vi "update_dict_HIS_DAT_update.vi"(8 "error in (no error)":errorcluster, 10 "type":string, 11 "dict of HIS IN":variant) -> (0 "error out":errorcluster, 3 "dict of HIS OUT":variant)   [LabVIEW 2015]
uses:
  cluster_template.ctl
  Classes/DATA/HIS/HIS.lvclass
  Classes/DATA/HIS/HIS.lvclass/HIS.ctl
  Classes/DATA/DATA.lvclass/DATA.ctl
  Classes/DATA/DATA.lvclass
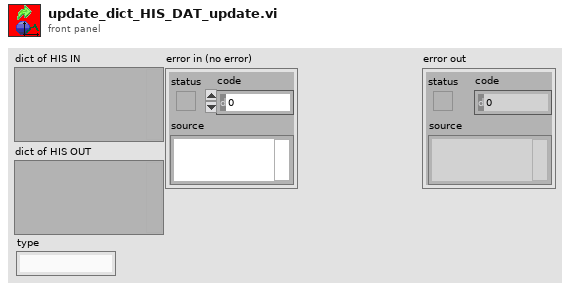
[diagram p1: front panel]
types:
  T1 = typedef "cluster_template.ctl" = cluster{"HIS.lvclass":refnum<class "HIS.lvclass">, "selector":refnum<vi>, "HIS graph":refnum<vi>, "DAT graph":refnum<vi>, "path":refnum<vi>, "path MAIN":refnum<vi>, "#":refnum<vi>, "unsel Graph":refnum<vi>, "DATgraph":refnum<vi>}
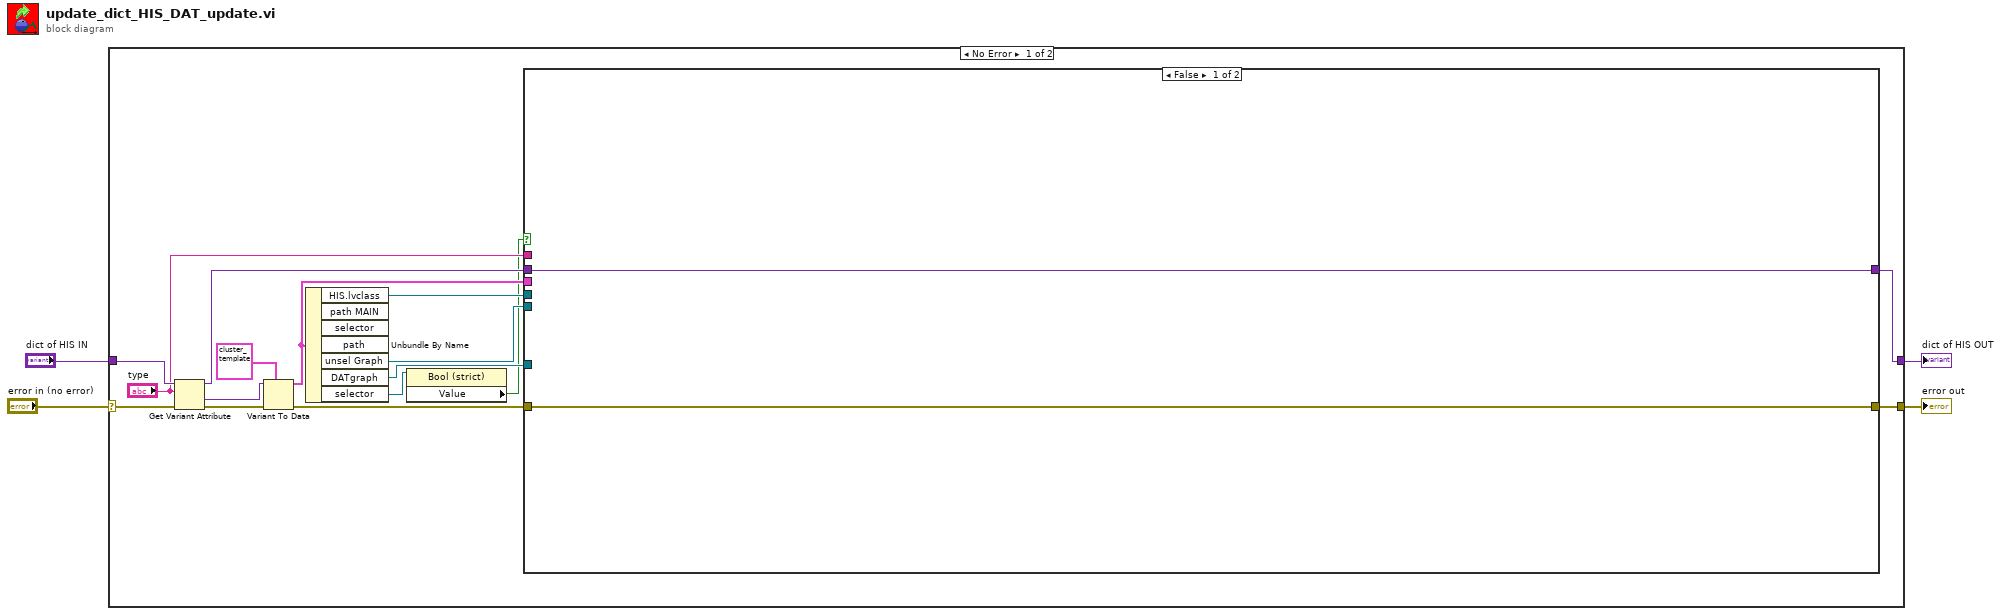
[diagram p0: block diagram]
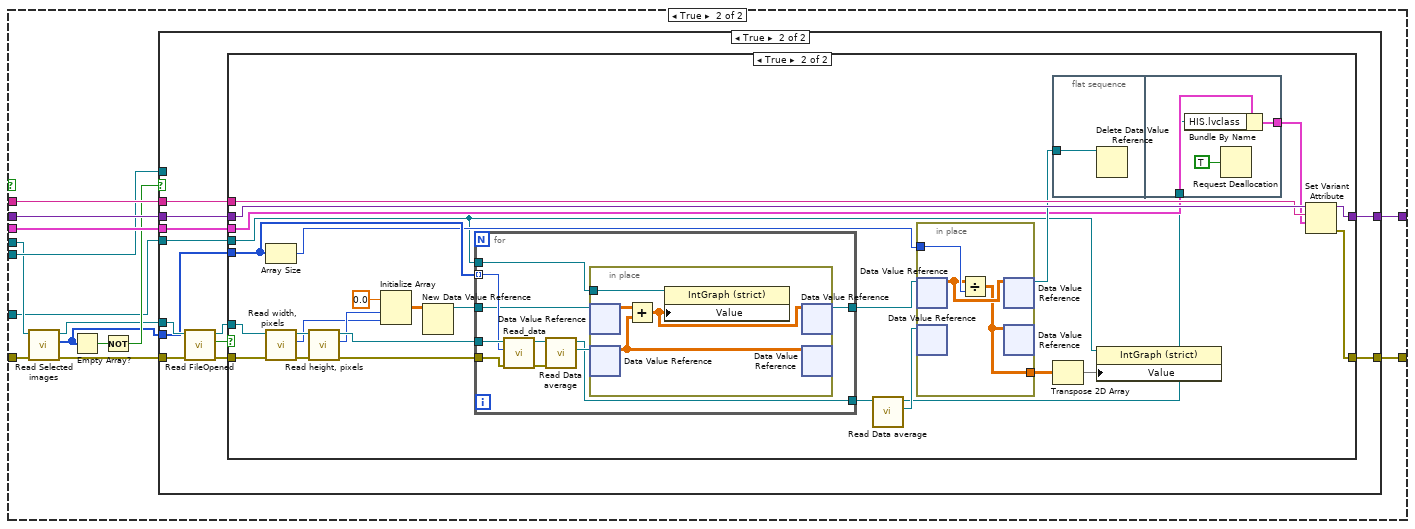
[diagram p2: hidden frame]
diagram:
  n1 = case shown="No Error" "error in (no error)" {
    selector: "error in (no error)" -> [w19 w103]
    tunnel: "dict of HIS IN" -> [w20 w102]
    tunnel: [w14 w102] -> w3
    tunnel: [w10 w103] -> w2
    frame No Error {
      n2 = Get Variant Attribute(Variant=w20, name="type", error in=w19) -> (duplicate Variant=w13:variant, value=w18:variant, error out=w17:errorcluster)  [unwired: 1 in, 1 out]
      n3 = Variant To Data(error in=w17, type=T1 {"HIS.lvclass"=refnum, "selector"=refnum, "HIS graph"=refnum, "DAT graph"=refnum, "path"=refnum, "path MAIN"=refnum, "#"=refnum, "unsel Graph"=refnum, "DATgraph"=refnum} ("output cluster"), Variant=w18) -> (data=w15:T1, error out=w9:errorcluster)
      n4 = Unbundle By Name(w15) -> ("HIS.lvclass"=w8:refnum<class "HIS.lvclass">, "unsel Graph"=w11:refnum<vi>, "DATgraph"=w7:refnum<vi>, "selector"=w6:refnum<vi>)  [unwired: 3 out]
      n5 = property class="Bool (strict)"(reference=w6) -> ("Value"=w5:bool)  [unwired: 1 in, 2 out]
      n6 = case shown="False" w5 {
        tunnel: w15 -> [_ w36]
        tunnel: [w22 w35] -> w14
        tunnel: w13 -> [w22 w34]
        tunnel: "type" -> [_ w33]
        tunnel: w11 -> [_ w32]
        tunnel: [w21 w31] -> w10
        tunnel: w9 -> [w21 w30]
        tunnel: w8 -> [_ w29]
        tunnel: w7 -> [_ w23]
        frame False {
        }
        frame True {
          n7 = call "Read Selected images.vi"("error in (no error)"=w30, "HIS in"=w29) -> ("error out"=w26:errorcluster, "Selected images"=w25:i32[], "HIS out"=w24:refnum<class "HIS.lvclass">)  [unwired: 7 in]
          n8 = Empty Array?(array=w25) -> (empty?=w28:bool)
          n9 = Not(x=w28) -> (.not. x?=w27:bool)
          n10 = case shown="True" w27 {
            tunnel: w36 -> [_ w41]
            tunnel: [w38 w50] -> w35
            tunnel: w34 -> [w38 w49]
            tunnel: w33 -> [_ w39]
            tunnel: w32 -> [_ _]
            tunnel: [w37 w48] -> w31
            tunnel: w26 -> [w37 w47]
            tunnel: w25 -> [_ w42]
            tunnel: w24 -> [_ w46]
            tunnel: w23 -> [_ w40]
            frame False {
            }
            frame True {
              n11 = call "Read FileOpened.vi"("error in (no error)"=w47, "DATA in"=w46) -> ("error out"=w45:errorcluster, "FileOpened"=w44:bool, "DATA out"=w43:refnum<class "HIS.lvclass">)  [unwired: 7 in]
              n12 = case shown="True" w44 {
                tunnel: [w52 w79] -> w50
                tunnel: w49 -> [w52 w78]
                tunnel: [w51 w77] -> w48
                tunnel: w45 -> [w51 w62]
                tunnel: w43 -> [_ w67]
                tunnel: w42 -> [_ w74]
                tunnel: w41 -> [_ w56]
                tunnel: w40 -> [_ w53]
                tunnel: w39 -> [_ w70]
                frame False {
                }
                frame True {
                  n13 = Array Size(array=w74) -> (size(s)=w73:i32)
                  n14 = call "Read width, pixels.vi"("error in (no error)"=w62, "DATA in"=w67) -> ("error out"=w63:errorcluster, "width, pixels"=w60:i32, "DATA out"=w66:refnum<class "HIS.lvclass">)  [unwired: 7 in]
                  n15 = call "Read height, pixels.vi"("error in (no error)"=w63, "DATA in"=w66) -> ("error out"=w64:errorcluster, "height, pixels"=w61:i32, "DATA out"=w65:refnum<class "HIS.lvclass">)  [unwired: 7 in]
                  n16 = Initialize Array(0.0 ("Numeric"), w61, w60) -> (w68:dbl[][])
                  n17 = New Data Value Reference(data value=w68) -> (data value reference=w76:refnum<data-value>)  [unwired: 1 in, 1 out]
                  n18 = for {
                    tunnel: w74 -> [w95] mode=indexing
                    tunnel: w65 -> [w96]
                    tunnel: w64 -> [w97]
                    tunnel: w76 -> [w91]
                    tunnel: [w90] -> w58
                    tunnel: [w89] -> w75
                    tunnel: w53 -> [w88]
                    n19 = call-dynamic "Read_data.vi"("error in (no error)"=w97, "#image"=w95, "HIS IN"=w96) -> ("error out"=w94:errorcluster, "HIS OUT"=w93:refnum<class "HIS.lvclass">)  [unwired: 7 in]
                    n20 = call "Read Data average.vi"("error in (no error)"=w94, "DATA in"=w93) -> ("Data average"=w92:refnum<data-value>, "DATA out"=w89:refnum<class "HIS.lvclass">)  [unwired: 7 in, 1 out]
                    n21 = in-place {
                      in-place-border: w88 -> [w99]
                      n22 = in-place-dvr #1(w91) -> (w101:dbl[][])  [unwired: 1 out]
                      n23 = in-place-dvr #2(w92) -> (w100:dbl[][])  [unwired: 1 out]
                      n24 = Add(x=w101, y=w100) -> (x+y=w98:dbl[][])
                      n25 = property class="IntGraph (strict)"(reference=w99, "Value"=w98) -> ()  [unwired: 1 in, 2 out]
                      n26 = in-place-dvr #1(w98) -> (w90:refnum<data-value>)  [unwired: 1 out]
                      n27 = in-place-dvr #2(w100) -> ()  [unwired: 2 out]
                    }
                  }
                  n28 = call "Read Data average.vi"("DATA in"=w75) -> ("Data average"=w59:refnum<data-value>, "DATA out"=w54:refnum<class "HIS.lvclass">)  [unwired: 8 in, 1 out]
                  n29 = in-place {
                    in-place-border: w73 -> [w82]
                    in-place-border: [w80] -> w72
                    n30 = in-place-dvr #3(w58) -> (w81:dbl[][])  [unwired: 1 out]
                    n31 = in-place-dvr #4(w59) -> ()  [unwired: 2 out]
                    n32 = Divide(x=w81, y=w82) -> (x/y=w80:dbl[][])
                    n33 = in-place-dvr #3(w81) -> (w57:refnum<data-value>)  [unwired: 1 out]
                    n34 = in-place-dvr #4(w80) -> ()  [unwired: 2 out]
                  }
                  n35 = flat-sequence {
                    tunnel: w57 -> [w83]
                    tunnel: w56 -> [w86]
                    tunnel: [w85] -> w55
                    tunnel: w54 -> [w84]
                    frame #0 {
                      n36 = Delete Data Value Reference(data value reference=w83) -> ()  [unwired: 1 in, 2 out]
                    }
                    frame #1 {
                      n37 = Bundle By Name(cluster=w86, "HIS.lvclass"=w84) -> (w85:T1)
                      n38 = Request Deallocation(TRUE ("flag")) -> ()
                    }
                  }
                  n39 = Transpose 2D Array(2D array=w72) -> (transposed array=w71:dbl[][])
                  n40 = property class="IntGraph (strict)"(reference=w53, "Value"=w71) -> ()  [unwired: 1 in, 2 out]
                  n41 = Set Variant Attribute(Variant=w78, name=w70, value=w55) -> (Variant out=w79:variant, error out=w77:errorcluster)  [unwired: 1 in, 1 out]
                }
              }
            }
          }
        }
      }
    }
    frame Error {
    }
  }
  "dict of HIS OUT" <- w3
  "error out" <- w2
